vi "Configure test.vi"(6 "Assert VI Path":path, 7 "Existing Queue Elements":string, 8 "error in (no error)":errorcluster, 11 "FP GTLT in":refnum<class "FP GTLT.lvclass">) -> (0 "error out":errorcluster, 3 "FP GTLT out":refnum<class "FP GTLT.lvclass">)   [LabVIEW 2018, in "FP GTLT.lvclass"]
uses:
  FP GTLT.lvclass
  f00565d1-d796-4672-996c-a63fd8227b78.vi
  <vilib>/JDP Science/JSONtext/Find Item.vi
  f00565d1-d796-4672-996c-a63fd8227b78.vi/55fc9789-8b6c-4666-8071-2353873a9f38.vi
  f00565d1-d796-4672-996c-a63fd8227b78.vi/29a07b18-84dd-499f-ab30-ed3b2ca4f395.vi
  <vilib>/JDP Science/JSONtext/String Subset.vi
  Test Class String IDs.vi
  <vilib>/JDP Science/JSONtext/Parsing/Parse Full Path or Item Name.vi
  <vilib>/JDP Science/JSONtext/Offset/Find Item Locations by Path.vi
  <vilib>/JDP Science/JSONtext/JSON text to Variant.vi
  <vilib>/JDP Science/JSONtext/Variant to JSON Text.vi
  <vilib>/JDP Science/JSONtext/Set Item.vi
  Floating Point.lvclass
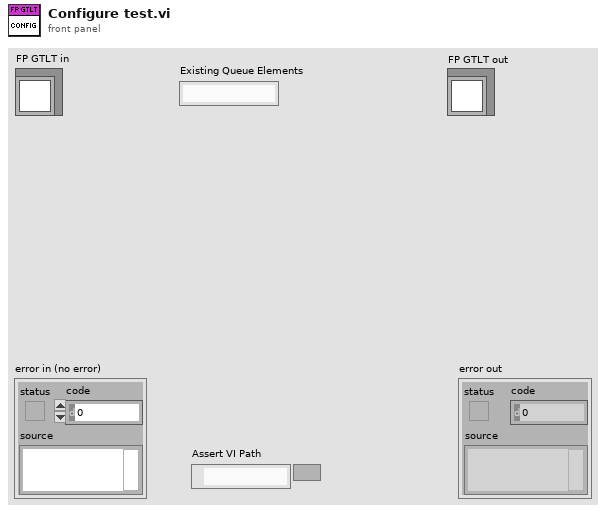
[diagram p1: front panel]
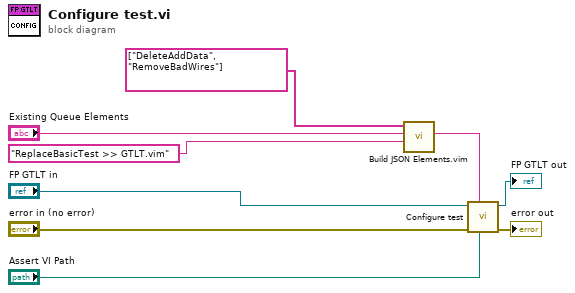
[diagram p0: block diagram]
diagram:
  n1 = call "Build JSON Elements.vim"("Append Element(s)"="ReplaceBasicTest >> GTLT.vim", "JSON Elements in ({})"="Existing Queue Elements", "Prepend Element(s)"=string[] ["DeleteAddData", "RemoveBadWires"]) -> ("JSON Elements out"=w2:string)  [unwired: 8 in]
  n2 = call-parent "Configure test.vi"("Assert VI Path"="Assert VI Path", "Existing Queue Elements"=w2, "error in (no error)"="error in (no error)", "Floating Point in"="FP GTLT in") -> ("error out"=→"error out":errorcluster, "Floating Point out"=→"FP GTLT out":refnum<class "FP GTLT.lvclass">)  [unwired: 6 in]
